vi "DSF.Shared.Configuration.Transfer Group.Get Transfer Configurations.vi"(11 "Transfer Group Configuration in":refnum<class "DSF.Shared.Configuration.Transfer Group.lvclass">) -> (2 "Transfer Configurations":refnum<class "DSF.Shared.Configuration.Transfer.lvclass">[](array[class]), 3 "Transfer Group Configuration out":refnum<class "DSF.Shared.Configuration.Transfer Group.lvclass">)   [LabVIEW 2017, in "DSF.Engine.lvlib" / "DSF.Shared.Configuration.Transfer Group.lvclass"]
uses:
  DSF.Shared.Configuration.Transfer Group.lvclass
  Transfer/DSF.Shared.Configuration.Transfer.lvclass
  DSF.Shared.Configuration.Transfer Group.lvclass/DSF.Shared.Configuration.Transfer Group.ctl
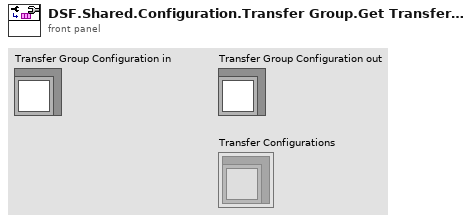
[diagram p1: front panel]
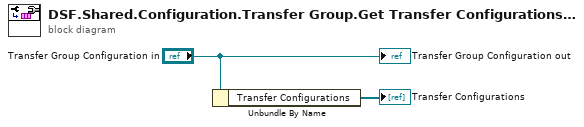
[diagram p0: block diagram]
diagram:
  n1 = Unbundle By Name("Transfer Group Configuration in") -> ("Transfer Configurations"=→"Transfer Configurations":refnum<class "DSF.Shared.Configuration.Transfer.lvclass">[])
  "Transfer Group Configuration out" <- "Transfer Group Configuration in"
